vi "Postflight Position.vi"(8 "error in (no error)":errorcluster) -> (0 "error out":errorcluster, 3 "function return":i32)   [LabVIEW 2020, in "ThorECU.lvlib"]
doc: "long PostflightPosition();"
uses:
  ThorECU.lvlib
  ThorECU.dll
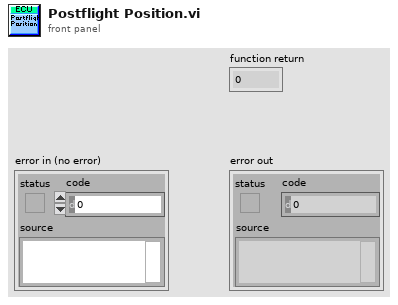
[diagram p1: front panel]
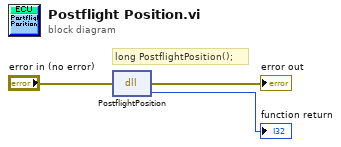
[diagram p0: block diagram]
diagram:
  # "long PostflightPosition();"
  n1 = dll-call lib="D:/software/TweezerTron Project/Instruments/Thorlabs/ECU_SDK/ThorECU.*" fn="PostflightPosition"(error in="error in (no error)") -> (error out=→"error out":errorcluster, →"function return":i32)  [unwired: 2 in, 1 out]
